vi "20181106.vi"() -> ()   [LabVIEW 2017]
panel:
  out "array w/ subset deleted":dbl[](array[numeric])
  out "ii":i32
  out "Waveform Chart":dbl(graph)
  in  "stop":bool
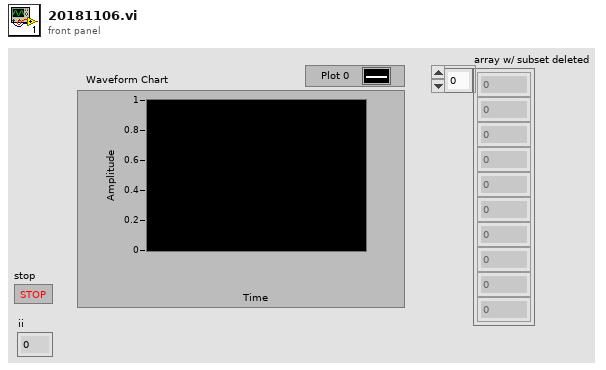
[diagram p1: front panel]
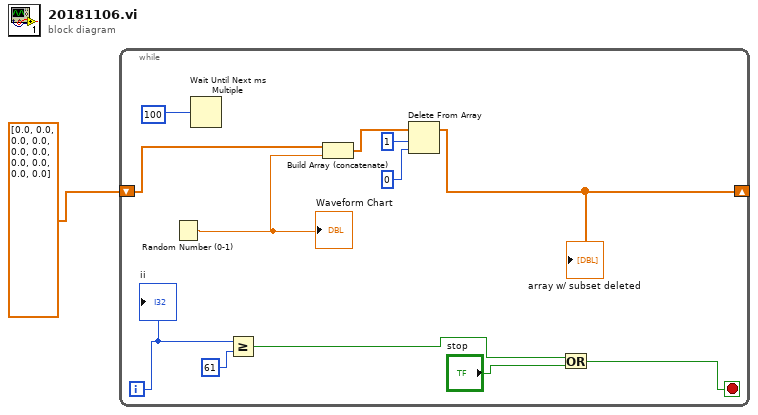
[diagram p0: block diagram]
diagram:
  n1 = while {
    shift-right: [w4] -> _
    shift-left: dbl[] [0.0, 0.0, 0.0, 0.0, 0.0, 0.0, 0.0, 0.0, 0.0, 0.0] ("Array") -> [w6]
    i -> [w8]
    stop <- w9 stop-if-true
    n2 = Random Number (0-1)() -> (number: 0 to 1=w7:dbl)
    "Waveform Chart" <- w7
    n3 = Wait Until Next ms Multiple(millisecond multiple=u32 100 ("millisecond timer value")) -> ()  [unwired: 1 out]
    n4 = Greater Or Equal?(x=w8, y=61) -> (x >= y?=w11:bool)
    n5 = Build Array (concatenate)(w6, w7) -> (w5:dbl[])
    n6 = Delete From Array(array=w5, length=1, index=0) -> (array with subset deleted=w4:dbl[])  [unwired: 1 out]
    "array w/ subset deleted" <- w4
    n7 = Or(x=w11, y="stop") -> (x .or. y?=w9:bool)
    "ii" <- w8
  }
